vi "Stop Core.vi"(10 "final error code":i32, 11 "[V] Sys Cfg Base in":refnum<class "[V] Sys Cfg Base.lvclass">) -> (3 "[V] Sys Cfg Base out":refnum<class "[V] Sys Cfg Base.lvclass">)   [LabVIEW 2023, in "[V] Sys Cfg Base.lvlib" / "[V] Sys Cfg Base.lvclass"]
doc: "(<B>Filename</B>: Actor Framework.lvlib:Actor.lvclass:Stop Core.vi)\n\nDefines what the actor does before it stops. Use the <B>final error code</B> input to determine whether the actor shut down in response to an error.\n\nBy default, this method passes the Stop message along to all auto-stop nested actors. A descendant class may override this method to define additional behavior, such as shutting down any processes the actor initiated in its override of the Actor Core method."
uses:
  [V] Sys Cfg Base.lvclass
  [V] Sys Cfg Base.lvclass/[V] Sys Cfg Base.ctl
  <vilib>/ActorFramework/Actor/Actor.lvclass
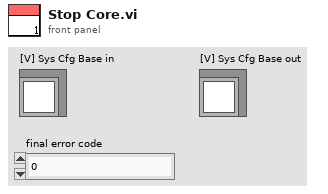
[diagram p1: front panel]
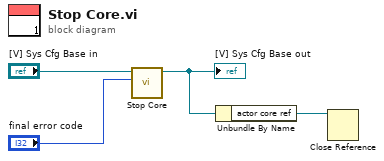
[diagram p0: block diagram]
diagram:
  n1 = call-parent "Stop Core.vi"("final error code"="final error code", "Actor in"="[V] Sys Cfg Base in") -> ("Actor out"=w2:refnum<class "[V] Sys Cfg Base.lvclass">)  [unwired: 9 in]
  "[V] Sys Cfg Base out" <- w2
  n2 = Unbundle By Name(w2) -> ("actor core ref"=w1:refnum<vi>)
  n3 = Close Reference(reference=w1) -> ()  [unwired: 1 in, 1 out]
